vi "OAT Coerce RPM Range.vi"(6 "speed profile":T2 {"speed [RPM]" format="%.2f"; "time [s]" format="%.2f"}, 7 "RPM range in":T1 {"Increment" format="%.2f"; "Maximum" format="%.2f"; "Minimum" format="%.2f"}) -> (1 "run up?":bool, 2 "total rpm":i32, 3 "RPM range out":T1 {"Increment" format="%.2f"; "Maximum" format="%.2f"; "Minimum" format="%.2f"})   [LabVIEW 2017]
uses:
  <vilib>/addons/Sound and Vibration/Order Analysis/Tach Process/SubVIs/speed profile.ctl
  <vilib>/addons/Sound and Vibration/Order Analysis/Tach Process/SoundVib_TachProcess.lvlib
panel:
  # "Coerce RPM Range"
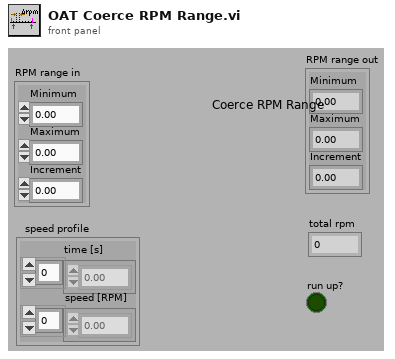
[diagram p1: front panel]
types:
  T1 = cluster{"Minimum":dbl, "Maximum":dbl, "Increment":dbl}
  T2 = typedef "SoundVib_TachProcess.lvlib/speed profile.ctl" = cluster{"time [s]":dbl[], "speed [RPM]":dbl[]}
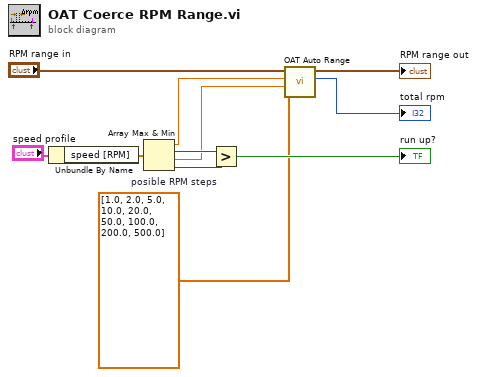
[diagram p0: block diagram]
diagram:
  w5 = dbl[] [1.0, 2.0, 5.0, 10.0, 20.0, 50.0, 100.0, 200.0, 500.0]  # posible RPM steps
  n1 = Unbundle By Name("speed profile") -> ("speed [RPM]"=w9:dbl[])
  n2 = Array Max & Min(array=w9) -> (max value=w4:dbl, max index (indices)=w8:i32, min value=w3:dbl, min index (indices)=w7:i32)
  n3 = Greater?(x=w8, y=w7) -> (0:→"run up?":bool)
  n4 = call <vilib>:"OAT Auto Range.vi"("posible increament"=w5, "lower limit"=w3, "upper limit"=w4, "range in"="RPM range in") -> ("total step"=→"total rpm":i32, "range out"=→"RPM range out":T1)  [unwired: 6 in]
